vi "Solve_weighted_AlphaT_7-30.vi"(1 "Complex |Epsilon/R|":dbl[][](array[numeric]), 2 "Alpha - Response Coefficients":cdb[][](array[numeric])) -> (0 "Alpha T '":cdb[][](array[numeric]))   [LabVIEW 2010]
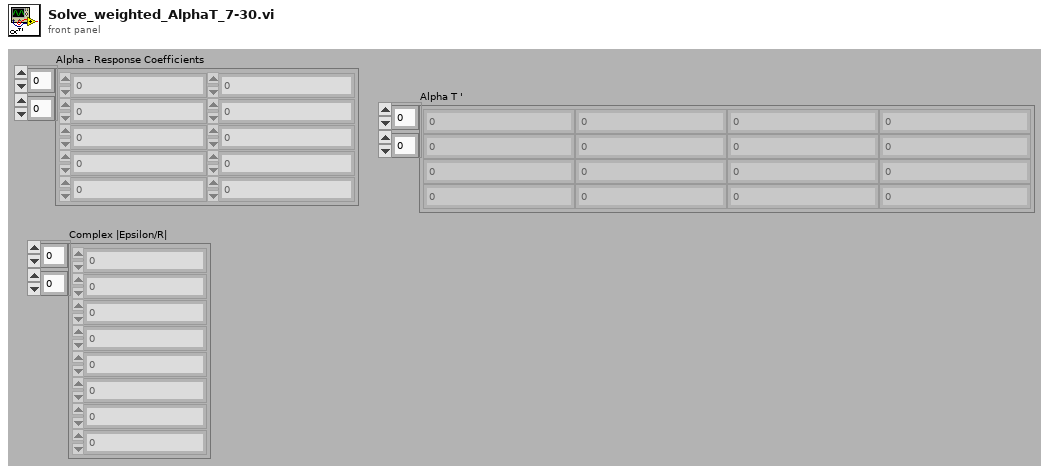
[diagram p1: front panel]
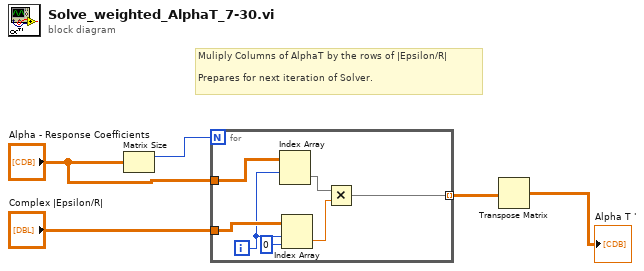
[diagram p0: block diagram]
diagram:
  # "Muliply Columns of AlphaT by the rows of |Epsilon/R|\n\nPrepares for next iteration of Solver."
  n1 = Matrix Size(0:"Alpha - Response Coefficients") -> (1:w1:i32)  [unwired: 1 out]
  n2 = for {
    N: w1 -> [_]
    tunnel: "Alpha - Response Coefficients" -> [w9]
    tunnel: "Complex |Epsilon/R|" -> [w12]
    tunnel: [w10] -> w3 mode=indexing
    i -> [w6]
    n3 = Index Array(array=w9, index (row)=w6) -> (element=w8:cdb[])  [unwired: 1 in]
    n4 = Index Array(array=w12, index (row)=w6, index (col)=0 ("disabled index (col)")) -> (element=w11:dbl)
    n5 = Multiply(x=w8, y=w11) -> (x*y=w10:cdb[])
  }
  n6 = Transpose Matrix(1:w3) -> (0:→"Alpha T '":cdb[][])
